vi "Open Bus Monitor.vi"(8 "error in (no error)":errorcluster, 11 "IMediator In":refnum<class "IMediator.lvclass">) -> (0 "error out":errorcluster, 3 "IMediator Out":refnum<class "IMediator.lvclass">)   [LabVIEW 2015, in "IMediator.lvlib" / "IMediator.lvclass"]
uses:
  IMediator.lvclass
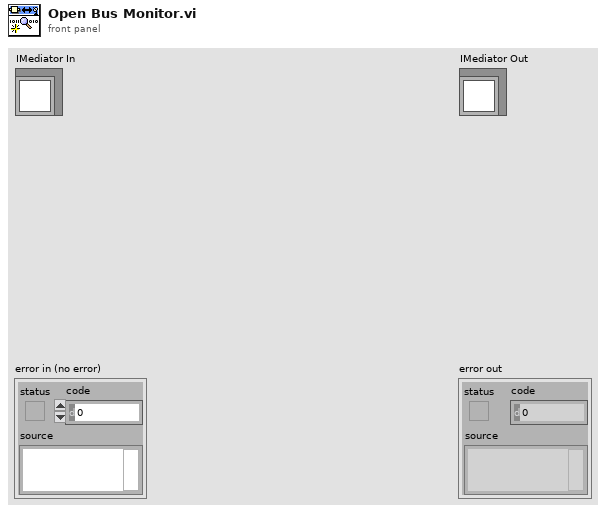
[diagram p1: front panel]
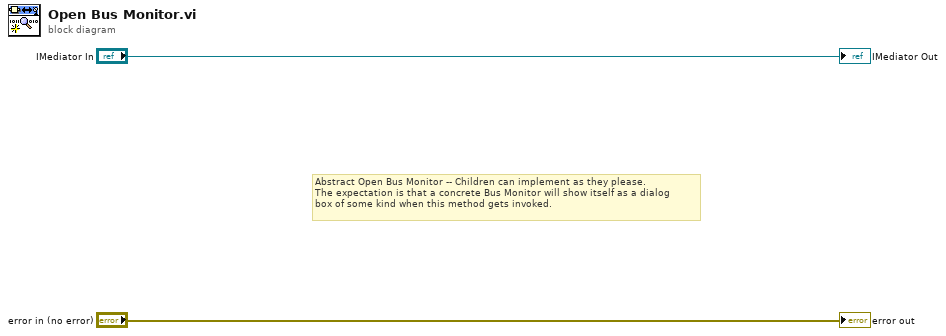
[diagram p0: block diagram]
diagram:
  # "Abstract Open Bus Monitor -- Children can implement as they please.\nThe expectation is that a concrete Bus Monitor will show itself as a dialog\nbox of some kind when this method gets invoked."
  "error out" <- "error in (no error)"
  "IMediator Out" <- "IMediator In"
